vi "Get Step Address(DC Manual).vi"(10 "Program Data.Mem Number":u32) -> (0 "Program Data.Start Address (Low)":string, 1 "Program Data.Start Address (Middle Low)":string, 2 "Program Data.Start Address (Middle High)":string, 3 "Program Data.Start Address (High)":string, 5 "Length (Low)":string, 7 "Length (High)":string)   [LabVIEW 2013]
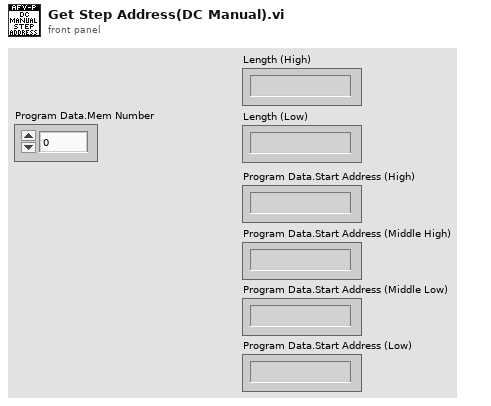
[diagram p1: front panel]
types:
  T1 = cluster{"Start Address (High)":string, "Start Address (Middle High)":string, "Start Address (Middle Low)":string, "Start Address (Low)":string, "Step Length":string, "Mem Number":u32, "Step Number":u32}
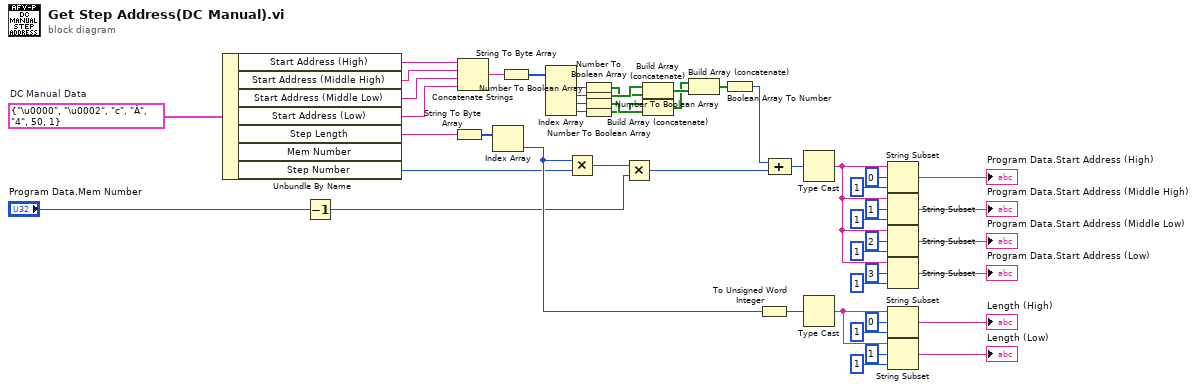
[diagram p0: block diagram]
diagram:
  w3 = T1 {"Start Address (High)"="\u0000", "Start Address (Middle High)"="\u0002", "Start Address (Middle Low)"="c", "Start Address (Low)"="Â", "Step Length"="4", "Mem Number"=50, "Step Number"=1}  # DC Manual Data
  n1 = Unbundle By Name(w3) -> ("Start Address (High)"=w9:string, "Start Address (Middle High)"=w8:string, "Start Address (Middle Low)"=w7:string, "Start Address (Low)"=w6:string, "Step Length"=w5:string, "Step Number"=w4:u32)  [unwired: 1 out]
  n2 = Decrement(x="Program Data.Mem Number") -> (x-1=w1:u32)
  n3 = String To Byte Array(string=w5) -> (unsigned byte array=w30:u8[])
  n4 = Concatenate Strings(w9, w8, w7, w6) -> (w40:string)
  n5 = Index Array(array=w30) -> (element=w10:u8)  [unwired: 1 in]
  n6 = String To Byte Array(string=w40) -> (unsigned byte array=w43:u8[])
  n7 = Index Array(array=w43) -> (element #1=w37:u8, element #2=w36:u8, element #3=w42:u8, element #4=w41:u8)  [unwired: 4 in]
  n8 = Multiply(x=w10, y=w4) -> (x*y=w12:u32)
  n9 = Number To Boolean Array(number=w37) -> (Boolean array=w34:bool[])
  n10 = Number To Boolean Array(number=w36) -> (Boolean array=w35:bool[])
  n11 = Number To Boolean Array(number=w42) -> (Boolean array=w39:bool[])
  n12 = Number To Boolean Array(number=w41) -> (Boolean array=w38:bool[])
  n13 = Multiply(x=w12, y=w1) -> (x*y=w18:u32)
  n14 = Build Array (concatenate)(w35, w34) -> (w33:bool[])
  n15 = Build Array (concatenate)(w38, w39) -> (w32:bool[])
  n16 = Build Array (concatenate)(w32, w33) -> (w31:bool[])
  n17 = Boolean Array To Number(Boolean array=w31) -> (number=w29:u32)
  n18 = To Unsigned Word Integer(number=w10) -> (unsigned 16bit integer=w11:u16)
  n19 = Compound Arithmetic op=ADD(w29, w18) -> (w19:u32)
  n20 = Type Cast(x=w19) -> (*(type *) &x=w20:string)  [unwired: 1 out]
  n21 = Type Cast(x=w11) -> (*(type *) &x=w13:string)  [unwired: 1 out]
  n22 = String Subset(string=w20, offset (0)=0, length (rest)=1 ("length (rest)")) -> (substring=→"Program Data.Start Address (High)":string)
  n23 = String Subset(string=w20, offset (0)=1, length (rest)=1 ("length (rest)")) -> (substring=→"Program Data.Start Address (Middle High)":string)
  n24 = String Subset(string=w20, offset (0)=2, length (rest)=1 ("length (rest)")) -> (substring=→"Program Data.Start Address (Middle Low)":string)
  n25 = String Subset(string=w20, offset (0)=3, length (rest)=1 ("length (rest)")) -> (substring=→"Program Data.Start Address (Low)":string)
  n26 = String Subset(string=w13, offset (0)=0, length (rest)=1 ("length (rest)")) -> (substring=→"Length (High)":string)
  n27 = String Subset(string=w13, offset (0)=1, length (rest)=1 ("length (rest)")) -> (substring=→"Length (Low)":string)
